vi "ConfigDM.vi"(7 "High Voltage":bool=TRUE, 8 "error in (no error)":errorcluster, 10 "Dev IDs":i32[](array[numeric]), 11 "Automation Refnum in":refnum<k7>) -> (0 "error out":errorcluster, 3 "Automation Refnum out":refnum<k7>)   [LabVIEW 2014]
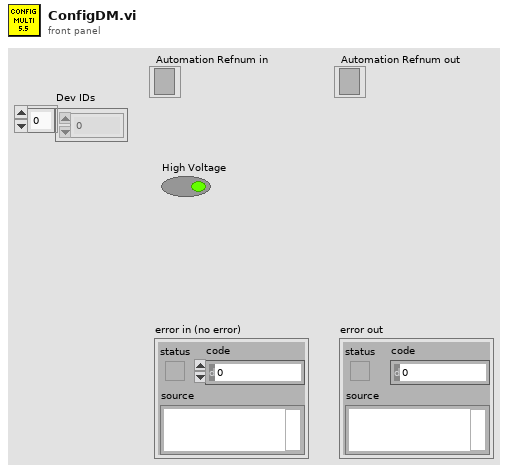
[diagram p1: front panel]
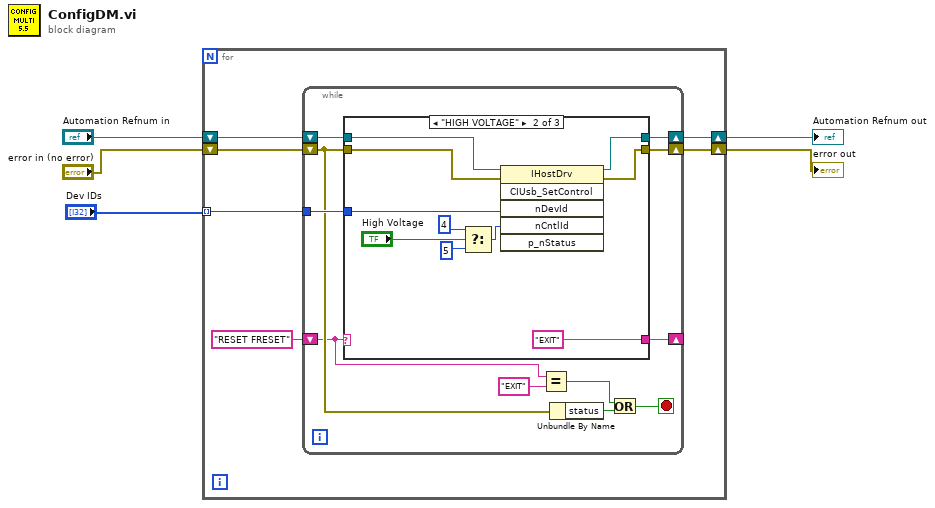
[diagram p0: block diagram]
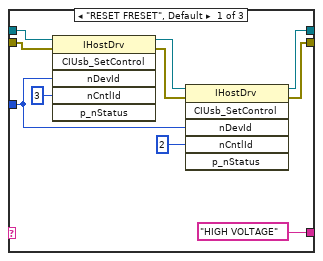
[diagram p2: hidden frame]
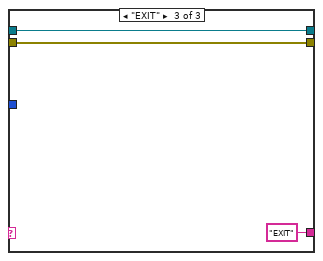
[diagram p3: hidden frame]
diagram:
  n1 = for {
    tunnel: "Dev IDs" -> [w6] mode=indexing
    shift-right: [w9] -> w4
    shift-left: "Automation Refnum in" -> [w7]
    shift-right: [w10] -> w5
    shift-left: "error in (no error)" -> [w8]
    n2 = while {
      tunnel: w6 -> [w22]
      shift-right: [w12] -> _
      shift-left: "RESET FRESET" -> [w17]
      shift-right: [w19] -> w10
      shift-left: w8 -> [w18]
      shift-right: [w20] -> w9
      shift-left: w7 -> [w21]
      stop <- w15 stop-if-true
      n3 = case shown="\"HIGH VOLTAGE\"" w17 {
        tunnel: w22 -> [w23 w42 _]
        tunnel: w21 -> [w32 w41 w45]
        tunnel: w18 -> [w31 w40 w44]
        tunnel: [w26 w39 w45] -> w20
        tunnel: [w24 w38 w44] -> w19
        tunnel: ["HIGH VOLTAGE" "EXIT" "EXIT"] -> w12
        frame "RESET FRESET", Default {
          n4 = invoke class="IHostDrv" method="CIUsb_SetControl"(reference=w32, error in=w31, "nDevId"=w23, "nCntlId"=3) -> (reference out=w27:refnum<k7>, error out=w25:errorcluster)  [unwired: 2 in, 4 out]
          n5 = invoke class="IHostDrv" method="CIUsb_SetControl"(reference=w27, error in=w25, "nDevId"=w23, "nCntlId"=2) -> (reference out=w26:refnum<k7>, error out=w24:errorcluster)  [unwired: 2 in, 4 out]
        }
        frame "HIGH VOLTAGE" {
          n6 = Select(t=4 ("nCntlId"), s="High Voltage", f=5 ("nCntlId")) -> (s? t:f=w33:i32)
          n7 = invoke class="IHostDrv" method="CIUsb_SetControl"(reference=w41, error in=w40, "nDevId"=w42, "nCntlId"=w33) -> (reference out=w39:refnum<k7>, error out=w38:errorcluster)  [unwired: 2 in, 4 out]
        }
        frame "EXIT" {
        }
      }
      n8 = Equal?(x=w17, y="EXIT") -> (x = y?=w13:bool)
      n9 = Unbundle By Name(w18) -> ("status"=w14:bool)
      n10 = Or(x=w13, y=w14) -> (x .or. y?=w15:bool)
    }
  }
  "error out" <- w5
  "Automation Refnum out" <- w4
